vi "SetPrice.vi"(8 "error in (no error)":errorcluster, 10 "Parcel Weight [kg]":dbl, 11 "Post in":refnum<class "Post.lvclass">) -> (0 "error out":errorcluster, 3 "Post out":refnum<class "Post.lvclass">)   [LabVIEW 2019, in "Post.lvclass"]
uses:
  Post.lvclass
  C:/Users/Extensa/Desktop/Fabryka/Fabryka Rozwiazanie/Delivery/Delivery/Delivery.lvclass
  Delivery/Delivery.lvclass/Delivery.ctl
  Delivery/Delivery.lvclass
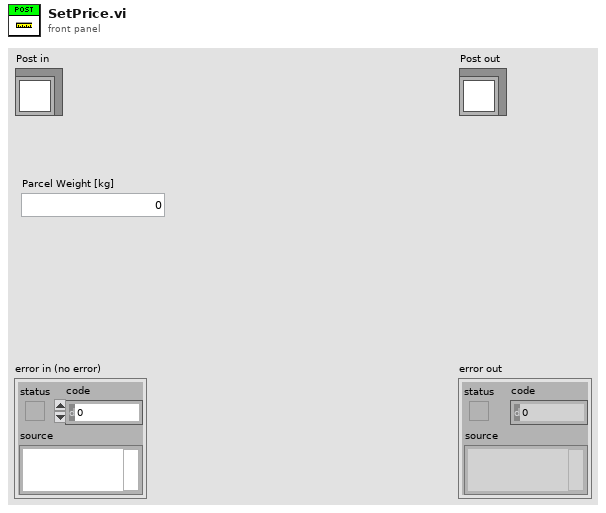
[diagram p1: front panel]
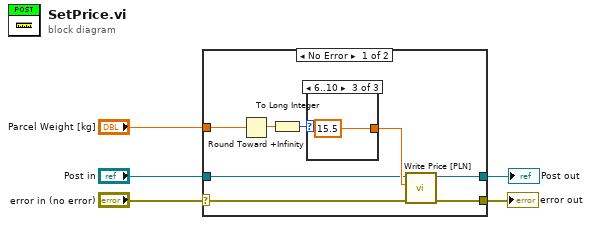
[diagram p0: block diagram]
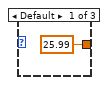
[diagram p2: hidden frame]
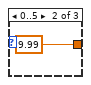
[diagram p3: hidden frame]
diagram:
  n1 = case shown="No Error" "error in (no error)" {
    selector: "error in (no error)" -> [w10 w18]
    tunnel: [w7 w18] -> w4
    tunnel: [w8 w17] -> w2
    tunnel: "Post in" -> [w9 w17]
    tunnel: "Parcel Weight [kg]" -> [w6 _]
    frame No Error {
      n2 = Round Toward +Infinity(x=w6) -> (ceil(x): smallest int >= x=w13:dbl)
      n3 = To Long Integer(number=w13) -> (32bit integer=w12:i32)
      n4 = case shown="6..10" w12 {
        tunnel: [25.99 9.99 15.5] -> w11
        frame Default {
        }
        frame 0..5 {
        }
        frame 6..10 {
        }
      }
      n5 = call "Write Price [PLN].vi"("error in (no error)"=w10, "Price [PLN]"=w11, "Delivery in"=w9) -> ("error out"=w7:errorcluster, "Delivery out"=w8:refnum<class "Post.lvclass">)  [unwired: 7 in]
    }
    frame Error {
    }
  }
  "error out" <- w4
  "Post out" <- w2
